vi "Actor Core.vi"(8 "error in":errorcluster, 11 "Orca-Flash 4.0 V2 in":refnum<class "Orca-Flash 4.0 V2.lvclass">) -> (0 "error out":errorcluster, 3 "Actor out":refnum<class "Actor.lvclass">)   [LabVIEW 2018, in "Orca-Flash 4.0 V2.lvlib" / "Orca-Flash 4.0 V2.lvclass"]
doc: "(<B>Filename</B>: Actor Framework.lvlib:Actor.lvclass:Actor Core.vi)\n\nReceives messages to the actor, reacts to them, and initiates any error handling that may shut the actor down.\n\nDescendant classes may override this VI to append parallel tasks for the actor to complete while it handles messages. Overrides use the Call Parent Method node."
uses:
  Orca-Flash 4.0 V2.lvclass
  C:/Program Files/National Instruments/LabVIEW 2018/vi.lib/ActorFramework/Actor/Actor.lvclass
  <vilib>/ActorFramework/Actor/Actor.lvclass
  <vilib>/ActorFramework/Actor/Actor.lvclass/Actor.ctl
  <vilib>/ActorFramework/Message Enqueuer/Message Enqueuer.lvclass/Message Enqueuer.ctl
  <vilib>/ActorFramework/Message Enqueuer/Init from Existing Queue.vi
  <vilib>/ActorFramework/Message Enqueuer/Enqueue.vi
  Orca-Flash 4.0 V2 Messages/Get Most Recent Frame (if active) Msg/Get Most Recent Frame (if active) Msg.lvclass
  C:/Program Files/National Instruments/LabVIEW 2018/vi.lib/ActorFramework/Message/Message.lvclass
  <vilib>/ActorFramework/Message Priority Queue/Priority Enqueue.vi
  <vilib>/ActorFramework/Message Enqueuer/Message Enqueuer.lvclass
  Camera/Camera.lvclass
panel:
  in  "Stop Button":bool
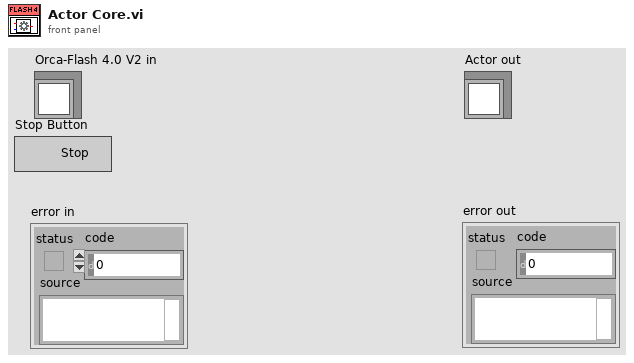
[diagram p1: front panel]
types:
  T1 = typedef "Semaphore RefNum" = refnum<k1>
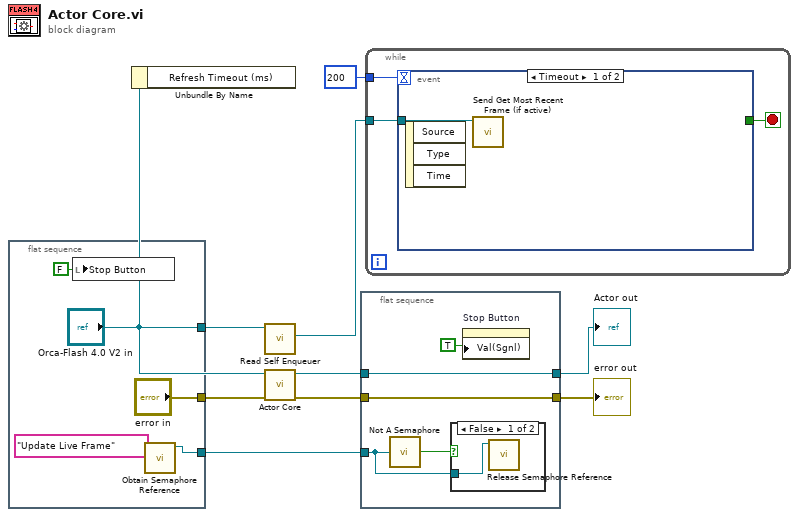
[diagram p0: block diagram]
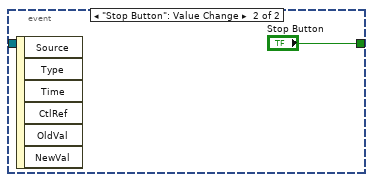
[diagram p3: hidden frame]
diagram:
  n1 = flat-sequence {
    tunnel: ["error in"] -> w9
    tunnel: ["Orca-Flash 4.0 V2 in"] -> w4
    tunnel: [w10] -> w2
    frame #0 {
      n2 = local write "Stop Button"(FALSE ("Stop Button")) -> ()
      n3 = call <vilib>:"Obtain Semaphore Reference.vi"("name (unnamed)"="Update Live Frame") -> ("semaphore"=w10:T1)  [unwired: 4 in, 2 out]
    }
  }
  n4 = Unbundle By Name(w4) -> ()  [unwired: 1 out]
  n5 = call <vilib>:"Read Self Enqueuer.vi"("Actor"=w4) -> ("Self Enqueuer"=w3:refnum<class "Message Enqueuer.lvclass">)  [unwired: 10 in]
  n6 = call-parent "Actor Core.vi"("error in"=w9, "Device in"=w4) -> ("error out"=w6:errorcluster, "Actor out"=w8:refnum<class "Actor.lvclass">)  [unwired: 8 in]
  n7 = flat-sequence {
    tunnel: w8 -> [w18]
    tunnel: [w18] -> w7
    tunnel: w6 -> [w17]
    tunnel: [w17] -> w5
    tunnel: w2 -> [w15]
    frame #0 {
      n8 = call <vilib>:"Not A Semaphore.vi"("semaphore"=w15) -> ("not a semaphore"=w16:bool)
      n9 = case shown="False" w16 {
        tunnel: w15 -> [w20 _]
        frame False {
          n10 = call <vilib>:"Release Semaphore Reference.vi"("semaphore"=w20) -> ()  [unwired: 9 in, 2 out]
        }
        frame True {
        }
      }
      n11 = property on="Stop Button" class="Bool (strict)"("Val(Sgnl)"=TRUE) -> ()  [unwired: 2 in, 2 out]
    }
  }
  n12 = while {
    tunnel: 200 ("Refresh Timeout (ms)") -> [w23]
    tunnel: w3 -> [w21]
    stop <- w22 stop-if-true
    n13 = event shown="[0] Timeout" {
      selector: _ -> [_ _]
      dyn-events: _ -> [_ _]
      timeout: w23 -> [_ _]
      tunnel: [_ "Stop Button"] -> w22
      tunnel: w21 -> [w24 _]
      event Timeout {
        n14 = event-data() -> ()  [unwired: 1 in, 3 out]
        n15 = call "Send Get Most Recent Frame (if active).vi"("Message Enqueuer"=w24) -> ()  [unwired: 9 in, 2 out]
      }
      event "Stop Button": Value Change {
        n16 = event-data() -> ()  [unwired: 1 in, 6 out]
      }
    }
  }
  "error out" <- w5
  "Actor out" <- w7
